vi "x-axis.vi"(8 "error in (no error)":errorcluster, 11 "Microwave Freq Scan in":refnum<class "Microwave Freq Scan.lvclass">) -> (0 "error out":errorcluster, 1 "Label":string, 2 "Unit":string, 3 "Microwave Freq Scan out":refnum<class "Microwave Freq Scan.lvclass">)   [LabVIEW 2017, in "Microwave Freq Scan.lvclass"]
uses:
  Microwave Freq Scan.lvclass
  Scanner/Scanner.lvclass
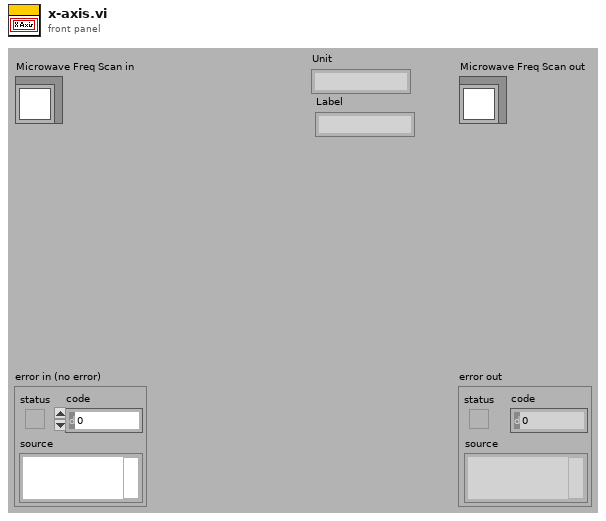
[diagram p1: front panel]
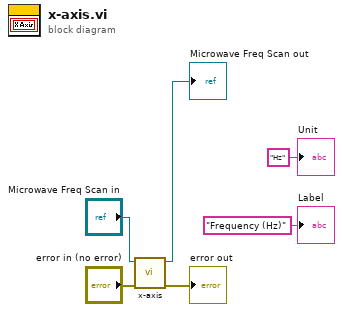
[diagram p0: block diagram]
diagram:
  n1 = call-parent "x-axis.vi"("error in (no error)"="error in (no error)", "Scanner in"="Microwave Freq Scan in") -> ("error out"=→"error out":errorcluster, "Scanner out"=→"Microwave Freq Scan out":refnum<class "Microwave Freq Scan.lvclass">)  [unwired: 6 in, 2 out]
  "Label" <- "Frequency (Hz)" ("Label")
  "Unit" <- "Hz" ("Unit")
